vi "Find Devices.vi"(8 "Error In":errorcluster) -> (0 "Error Out":errorcluster, 2 "Num Devices":i32, 3 "Device Names":string[](array[string]))   [LabVIEW 2011]
uses:
  <vilib>/LabVIEW Hacker/Adept/Private/DMGR/DMGR.lvlib
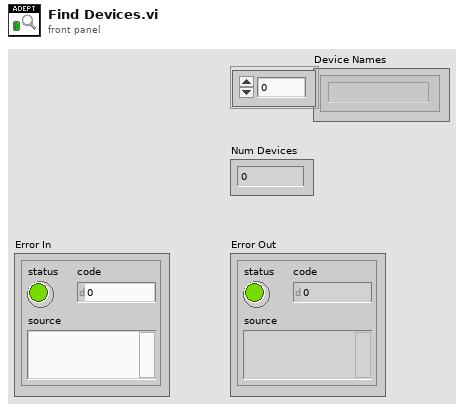
[diagram p1: front panel]
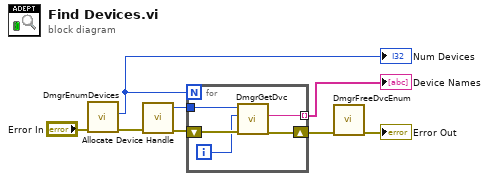
[diagram p0: block diagram]
diagram:
  n1 = call <vilib>:"DmgrEnumDevices.vi"("Error In"="Error In") -> ("Error Out"=w8:errorcluster, "Num Devices"=w5:i32)  [unwired: 9 in]
  "Num Devices" <- w5
  n2 = call <vilib>:"Allocate Device Handle.vi"("Error In"=w8) -> ("Error Out"=w7:errorcluster, "Device Handle"=w6:u64)  [unwired: 9 in]
  n3 = for {
    N: w5 -> [_]
    tunnel: w6 -> [w12]
    tunnel: [w11] -> w1 mode=indexing
    shift-right: [w10] -> w2
    shift-left: w7 -> [w13]
    i -> [w9]
    n4 = call <vilib>:"DmgrGetDvc.vi"("Error In"=w13, "Device Number"=w9, "Device Handle"=w12) -> ("Error Out"=w10:errorcluster, "Name"=w11:string)  [unwired: 4 in, 3 out]
  }
  "Device Names" <- w1
  n5 = call <vilib>:"DmgrFreeDvcEnum.vi"("Error In"=w2) -> ("Error Out"=→"Error Out":errorcluster)  [unwired: 10 in]
